vi "setCommunicator.vi"(10 "Communicator":refnum<class "Communicator.lvclass">, 11 "Telemetry in":refnum<class "Telemetry.lvclass">) -> (3 "Telemetry out":refnum<class "Telemetry.lvclass">)   [LabVIEW 2016, in "Telemetry.lvclass"]
uses:
  Telemetry.lvclass
  Communicator/Communicator/Communicator.lvclass
  Telemetry.lvclass/Telemetry.ctl
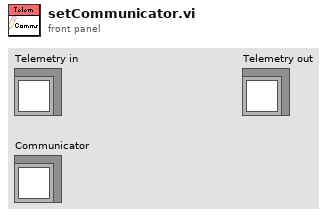
[diagram p1: front panel]
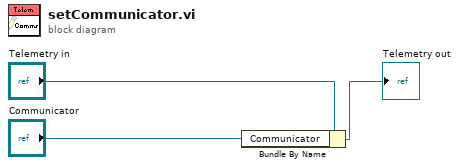
[diagram p0: block diagram]
diagram:
  n1 = Bundle By Name(cluster="Telemetry in", "Communicator"="Communicator") -> (→"Telemetry out":refnum<class "Telemetry.lvclass">)
